vi "Simulate Waveguide.vi"(8 "error in (no error)":errorcluster, 9 "Waveguide Cluster":T1={"Vsource Index"=0, "Vsg Index"=1, "V+"=0, "V-"=0}, 10 "AO []":waveform(dbl)[](array[waveform]), 11 "Instrument.Lockin.lvlib:Instrument.DAQ.lvclass":refnum<class "Instrument.DAQ.lvclass">) -> (0 "error out":errorcluster, 2 "AI []":waveform(dbl)[](array[waveform]), 3 "Instrument.Lockin.lvlib:Instrument.DAQ.lvclass":refnum<class "Instrument.DAQ.lvclass">)   [LabVIEW 2019, in "Instrument.Lockin.lvlib" / "Instrument.DAQ.lvclass"]
uses:
  Instrument.DAQ.lvclass
  Waveguide Model/Waveguide Model--Cluster.ctl
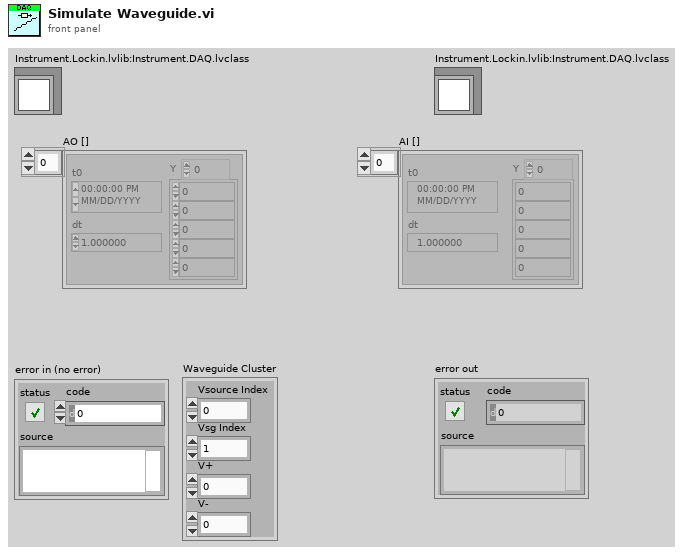
[diagram p1: front panel]
types:
  T1 = typedef "Instrument.Lockin.lvlib/Instrument.DAQ.lvclass/Waveguide Model--Cluster.ctl" = cluster{"Vsource Index":i32, "Vsg Index":i32, "V+":i32, "V-":i32}
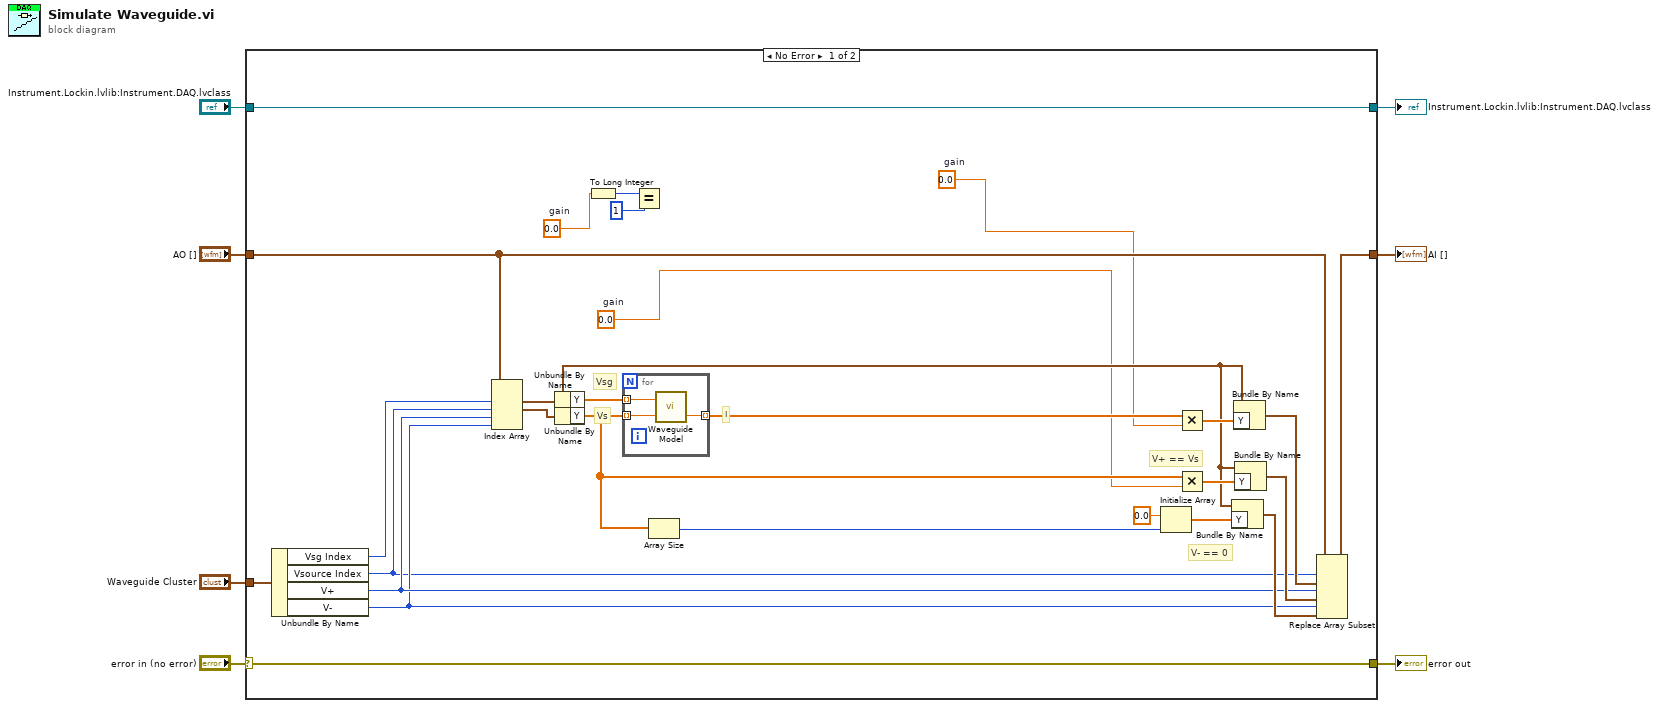
[diagram p0: block diagram]
diagram:
  n1 = case shown="No Error" "error in (no error)" {
    selector: "error in (no error)" -> [w11 w38]
    tunnel: "Waveguide Cluster" -> [w32 _]
    tunnel: [w29 w39] -> w6
    tunnel: [w11 w38] -> w4
    tunnel: [w13 w40] -> w3
    tunnel: "Instrument.Lockin.lvlib:Instrument.DAQ.lvclass" -> [w13 w40]
    tunnel: "AO []" -> [w30 w39]
    frame No Error {
      w8 = 0.0  # gain
      w9 = 0.0  # gain
      w10 = 0.0  # gain
      # "V- == 0"
      # "V+ == Vs"
      # "I"
      # "Vs"
      # "Vsg"
      n2 = Unbundle By Name(w32) -> ("Vsg Index"=w28:i32, "Vsource Index"=w12:i32, "V+"=w17:i32, "V-"=w16:i32)
      n3 = Index Array(array=w30, index #1=w28, index #2=w12, index #3=w17, index #4=w16) -> (element #1=w19:waveform(dbl), element #2=w27:waveform(dbl))  [unwired: 2 out]
      n4 = Unbundle By Name(w19) -> ("Y"=w31:dbl[])
      n5 = Unbundle By Name(w27) -> ("Y"=w23:dbl[])
      n6 = To Long Integer(number=w9) -> (32bit integer=w15:i32)
      n7 = for {
        tunnel: w23 -> [w37] mode=indexing
        tunnel: w31 -> [w36] mode=indexing
        tunnel: [w35] -> w34 mode=indexing
        n8 = call "Waveguide Model.vi"("Vs (V)"=w37, "Vsg (V)"=w36) -> ("I[Vsg] (A)"=w35:dbl)  [unwired: 1 out]
      }
      n9 = Equal?(x=w15, y=1 ("x")) -> ()  [unwired: 1 out]
      n10 = Array Size(array=w23) -> (size(s)=w22:i32)
      n11 = Initialize Array(0.0 ("y"), w22) -> (w20:dbl[])
      n12 = Multiply(x=w34, y=w8) -> (x*y=w33:dbl[])
      n13 = Multiply(x=w23, y=w10) -> (x*y=w25:dbl[])
      n14 = Bundle By Name(cluster=w19, "Y"=w20) -> (w18:waveform(dbl))
      n15 = Bundle By Name(cluster=w19, "Y"=w33) -> (w26:waveform(dbl))
      n16 = Bundle By Name(cluster=w19, "Y"=w25) -> (w24:waveform(dbl))
      n17 = Replace Array Subset(array=w30, new element #1=w26, index #1=w12, new element #2=w24, index #2=w17, new element #3=w18, index #3=w16) -> (w29:waveform(dbl)[])
    }
    frame Error {
    }
  }
  "error out" <- w4
  "Instrument.Lockin.lvlib:Instrument.DAQ.lvclass" <- w3
  "AI []" <- w6
